vi "Start_Initial.vi"(8 "error in (no error)":errorcluster, 11 "Reference":T1) -> (0 "error out":errorcluster, 3 "dup Reference":T1)   [LabVIEW 2020]
uses:
  Button_Reference.ctl
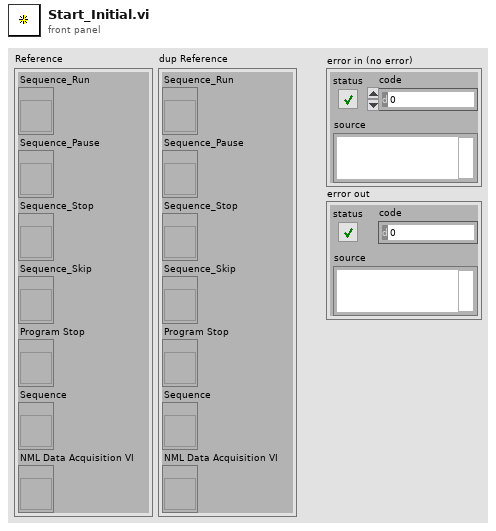
[diagram p1: front panel]
types:
  T1 = typedef "Button_Reference.ctl" = cluster{"Sequence_Run":refnum<vi>, "Sequence_Pause":refnum<vi>, "Sequence_Stop":refnum<vi>, "Sequence_Skip":refnum<vi>, "Program Stop":refnum<vi>, "Sequence":refnum<vi>, "NML Data Acquisition VI":refnum<vi>}
  T2 = enum8{"Enabled", "Disabled", "Disabled and Grayed Out"}
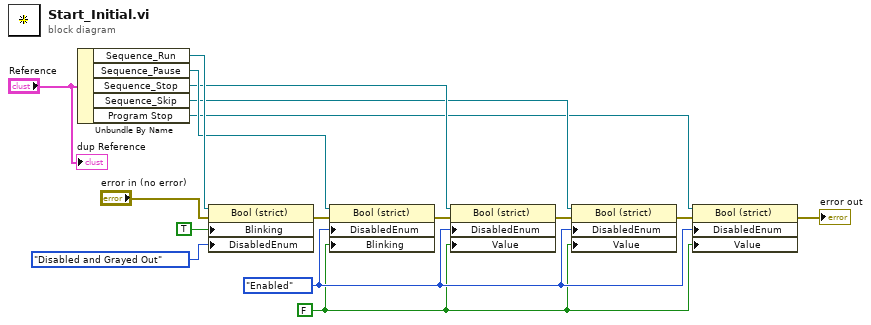
[diagram p0: block diagram]
diagram:
  w2 = FALSE
  w8 = T2."Enabled" ("Disabled")
  n1 = Unbundle By Name("Reference") -> ("Sequence_Run"=w7:refnum<vi>, "Sequence_Pause"=w6:refnum<vi>, "Sequence_Stop"=w5:refnum<vi>, "Sequence_Skip"=w4:refnum<vi>, "Program Stop"=w3:refnum<vi>)
  n2 = property on="Property Node" class="Bool (strict)"(reference=w7, error in="error in (no error)", "Blinking"=TRUE, "DisabledEnum"=T2."Disabled and Grayed Out" ("Disabled")) -> (error out=w14:errorcluster)  [unwired: 1 out]
  n3 = property on="Property Node" class="Bool (strict)"(reference=w6, error in=w14, "DisabledEnum"=w8, "Blinking"=w2) -> (error out=w15:errorcluster)  [unwired: 1 out]
  n4 = property on="Property Node" class="Bool (strict)"(reference=w5, error in=w15, "DisabledEnum"=w8, "Value"=w2) -> (error out=w16:errorcluster)  [unwired: 1 out]
  n5 = property on="Property Node" class="Bool (strict)"(reference=w4, error in=w16, "DisabledEnum"=w8, "Value"=w2) -> (error out=w9:errorcluster)  [unwired: 1 out]
  n6 = property on="Property Node" class="Bool (strict)"(reference=w3, error in=w9, "DisabledEnum"=w8, "Value"=w2) -> (error out=→"error out":errorcluster)  [unwired: 1 out]
  "dup Reference" <- "Reference"
